vi "AudioStreamer.Set Config.vi"(0 "Fs (Hz)":dbl, 5 "device":string, 11 "error in (no error)":errorcluster) -> (15 "error out":errorcluster)   [LabVIEW 2020]
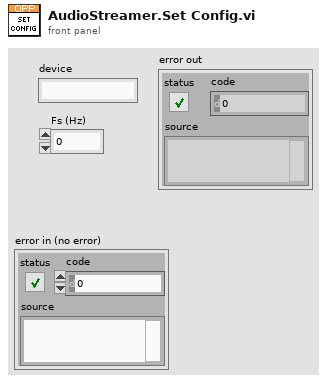
[diagram p1: front panel]
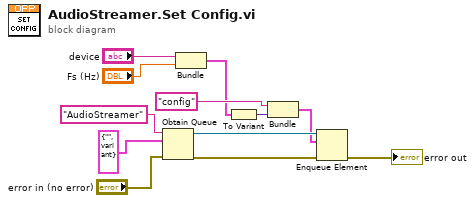
[diagram p0: block diagram]
diagram:
  n1 = Obtain Queue(name (unnamed)="AudioStreamer", element data type=cluster{string, variant} {"", variant}, error in (no error)="error in (no error)") -> (queue out=w9:refnum<queue>, error out=w10:errorcluster)  [unwired: 2 in, 1 out]
  n2 = Bundle("device"="device", "Fs (Hz)"="Fs (Hz)") -> (w2:cluster{"device":string, "Fs (Hz)":dbl})  [unwired: 1 in]
  n3 = To Variant(anything=w2) -> (Variant=w7:variant)
  n4 = Bundle("config", "Variant"=w7) -> (w5:cluster{string, "Variant":variant})  [unwired: 1 in]
  n5 = Enqueue Element(queue=w9, element=w5, error in (no error)=w10) -> (error out=→"error out":errorcluster)  [unwired: 1 in, 2 out]
